vi "Write Channels.vi"(8 "error in (no error)":errorcluster, 10 "Channels":T1, 11 "RSI Module in":refnum<class "RSI Module.lvclass">) -> (0 "error out":errorcluster, 3 "RSI Module out":refnum<class "RSI Module.lvclass">)   [LabVIEW 2017, in "Modules.lvlib" / "RSI Module.lvclass"]
uses:
  RSI Module.lvclass
  Channels.ctl
  Channel Type.ctl
  RSI Module.lvclass/RSI Module.ctl
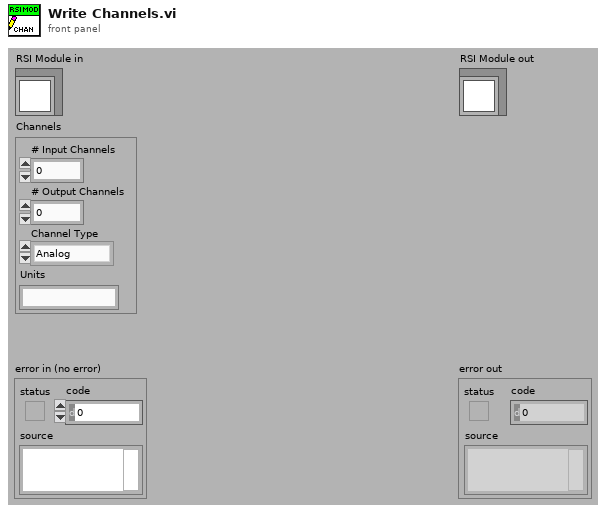
[diagram p1: front panel]
types:
  T1 = typedef "Modules.lvlib/RSI Module.lvclass/Channels.ctl" = cluster{"# Input Channels":i32, "# Output Channels":i32, "Channel Type":T2, "Units":string}
  T2 = typedef "Modules.lvlib/RSI Module.lvclass/Channel Type.ctl" = enum16{"Analog", "Digital"}
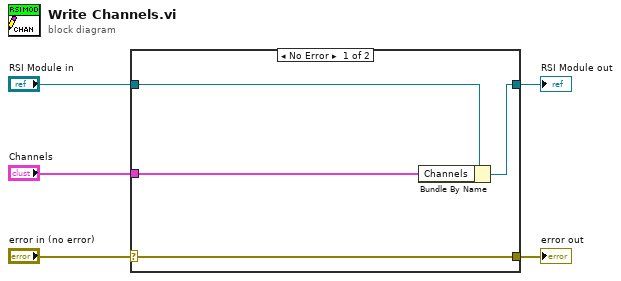
[diagram p0: block diagram]
diagram:
  n1 = case shown="No Error" "error in (no error)" {
    selector: "error in (no error)" -> [w9 w10]
    tunnel: [w9 w10] -> w4
    tunnel: [w7 w11] -> w2
    tunnel: "RSI Module in" -> [w8 w11]
    tunnel: "Channels" -> [w6 _]
    frame No Error {
      n2 = Bundle By Name(cluster=w8, "Channels"=w6) -> (w7:refnum<class "RSI Module.lvclass">)
    }
    frame Error {
    }
  }
  "error out" <- w4
  "RSI Module out" <- w2
